vi "Utilizarea ferestrelor de timp pentru netezire.vi"() -> ()   [LabVIEW 2011]
uses:
  <vilib>/Analysis/4window.llb/Hanning Window (DBL).vi
  <vilib>/Analysis/NI_AALBase.lvlib
  <vilib>/Analysis/NI_AALPro.lvlib
panel:
  in  "No. of Cycles":dbl
  in  "Amplitude":dbl
  out "Spectrum of Windowed Signal":dbl[](graph)
  out "Spectrum of Original Signal":dbl[](graph)
  out "Windowed Signal":dbl[](graph)
  out "Original Signal":dbl[](graph)
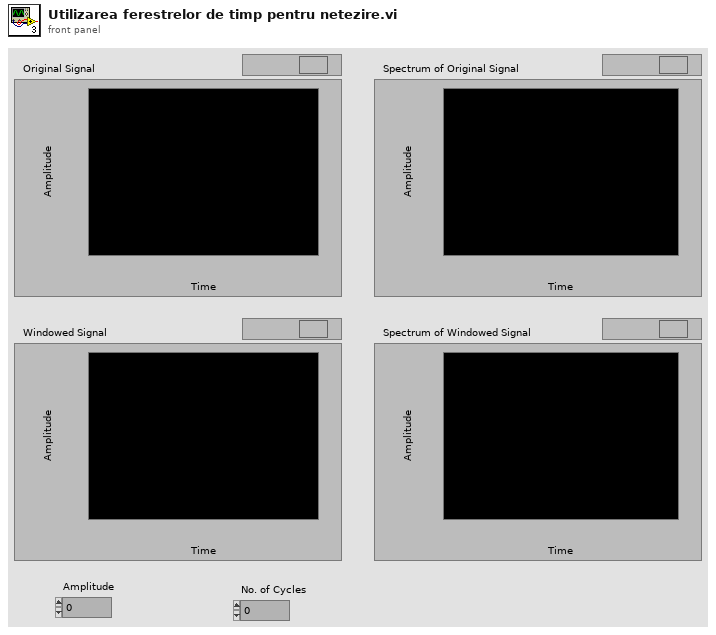
[diagram p1: front panel]
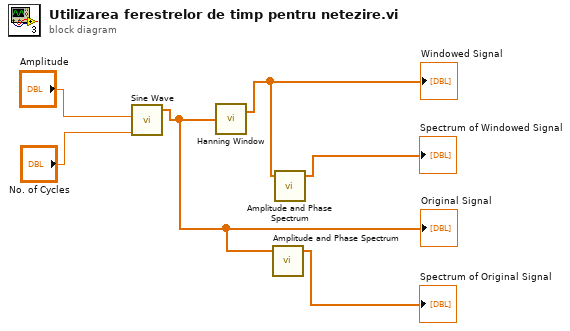
[diagram p0: block diagram]
diagram:
  n1 = call <vilib>:"Sine Wave.vi"("amplitude"="Amplitude", "phase in"="No. of Cycles") -> ("sine wave"=w2:dbl[])  [unwired: 3 in, 2 out]
  "Original Signal" <- w2
  n2 = call-poly <vilib>:"Hanning Window.vi"("X"=w2) -> ("Windowed X"=w4:dbl[])  [unwired: 1 out]
  "Windowed Signal" <- w4
  n3 = call <vilib>:"Amplitude and Phase Spectrum.vi"("Signal (V)"=w2) -> ("Amp Spectrum Mag (Vrms)"=→"Spectrum of Original Signal":dbl[])  [unwired: 2 in, 2 out]
  n4 = call <vilib>:"Amplitude and Phase Spectrum.vi"("Signal (V)"=w4) -> ("Amp Spectrum Mag (Vrms)"=→"Spectrum of Windowed Signal":dbl[])  [unwired: 2 in, 2 out]
